vi "Set Knock Cylinder Properties.vi"(8 "error in (no error)":errorcluster, 10 "cylinder":T1={"Name"="", "Bitfile name"="", "Probability"=0.0, "Amplitude"=-90.0, "Angle"=0.0}, 11 "Item Ref in":T2 format="%.0x") -> (0 "error out":errorcluster, 2 "failed":bool, 3 "Item Ref out":T2 format="%.0x")   [LabVIEW 2017, in "Engine Simulation Toolkit System Explorer.lvlib"]
uses:
  Engine Simulation Toolkit System Explorer.lvlib
  <vilib>/NI Veristand/Custom Device API/Custom Device Item Ref.ctl
  Knock Cylinder.ctl
  Shared/Properties.vi
  <vilib>/NI Veristand/Custom Device Tools/Custom Device Utility Library/NI VeriStand - Search for Item by Property.vi
  Shared/Constants and GUIDs.vi
  Shared/Engine Simulation Toolkit Shared.lvlib
  <vilib>/NI Veristand/Custom Device Tools/Custom Device Utility Library/Custom Device Utility Library.lvlib
  <vilib>/NI Veristand/Custom Device API/Custom Device API.lvlib
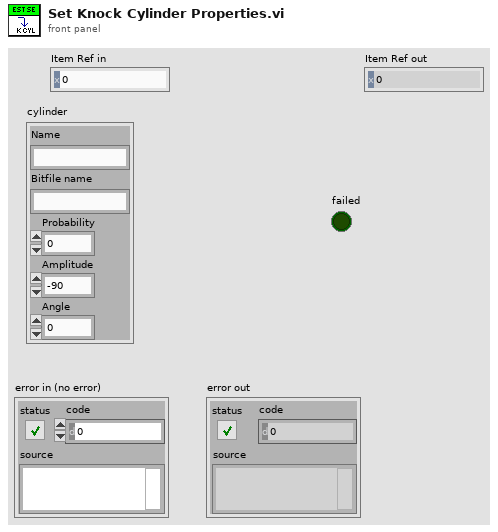
[diagram p1: front panel]
types:
  T1 = typedef "Engine Simulation Toolkit System Explorer.lvlib/Knock Cylinder.ctl" = cluster{"Name":string, "Bitfile name":string, "Probability":dbl, "Amplitude":dbl, "Angle":dbl}
  T2 = typedef "Custom Device API.lvlib/Custom Device Item Ref.ctl" = u64
  T3 = typedef "Engine Simulation Toolkit Shared.lvlib/Channel.ctl" = cluster{"Name":string, "Units":string, "Default":dbl, "Description":string, "Scalable":bool}
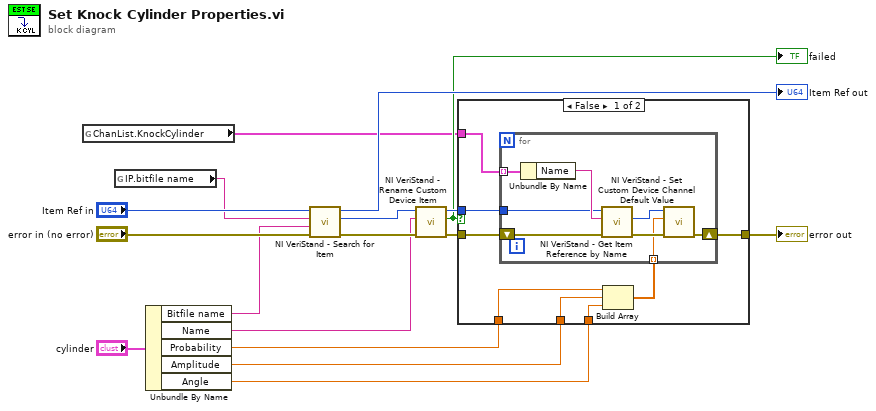
[diagram p0: block diagram]
diagram:
  n1 = global read "Constants and GUIDs.vi" "ChanList.KnockCylinder"() -> (w2:T3[])
  n2 = global read "Properties.vi" "IP.bitfile name"() -> (w8:string)
  n3 = Unbundle By Name("cylinder") -> ("Bitfile name"=w9:string, "Name"=w4:string, "Probability"=w1:dbl, "Amplitude"=w11:dbl, "Angle"=w10:dbl)
  n4 = call-poly <vilib>:"NI VeriStand - Search for Item.vi"("error in"="error in (no error)", "Property Value"=w9, "Property Name"=w8, "Section Ref in"="Item Ref in") -> ("error out"=w14:errorcluster, "Item Ref"=w6:T2, "Section Ref out"=→"Item Ref out":T2)  [unwired: 4 in, 1 out]
  n5 = call <vilib>:"NI VeriStand - Rename Custom Device Item.vi"("error in (no error)"=w14, "New Name"=w4, "Item Ref in"=w6) -> ("error out"=w7:errorcluster, "Request invalid?"=w3:bool, "Item Ref out"=w5:T2)  [unwired: 6 in]
  "failed" <- w3
  n6 = case shown="False" w3 {
    tunnel: [w24 w34] -> w16
    tunnel: w11 -> [w22 _]
    tunnel: w10 -> [w21 _]
    tunnel: w7 -> [w25 w34]
    tunnel: w5 -> [w19 _]
    tunnel: w2 -> [w23 _]
    tunnel: w1 -> [w18 _]
    frame False {
      n7 = Build Array(w18, w22, w21) -> (w20:dbl[])
      n8 = for {
        shift-right: [w27] -> w24
        shift-left: w25 -> [w33]
        tunnel: w23 -> [w32] mode=indexing
        tunnel: w19 -> [w30]
        tunnel: w20 -> [w26] mode=indexing
        n9 = Unbundle By Name(w32) -> ("Name"=w31:string)
        n10 = call <vilib>:"NI VeriStand - Get Item Reference by Name.vi"("error in (no error)"=w33, "Item Name"=w31, "Parent Ref in"=w30) -> ("error out"=w29:errorcluster, "Item Ref"=w28:T2)  [unwired: 5 in, 2 out]
        n11 = call <vilib>:"NI VeriStand - Set Custom Device Channel Default Value.vi"("error in (no error)"=w29, "Default Value"=w26, "Channel Ref in"=w28) -> ("error out"=w27:errorcluster)  [unwired: 7 in, 1 out]
      }
    }
    frame True {
    }
  }
  "error out" <- w16
